vi "Teleop.vi"(10 "Match Info":T1={"Autonomous Elapsed Seconds"=0.0, "TeleOp Elapsed Seconds"=0.0, "Disabled Elapsed Seconds"=0.0, "Visited Autonomous"=FALSE, "Visited TeleOp"=FALSE, "Visited Disabled"=FALSE, "Autonomous Settings"={"Autonomous Style"=enum."Independent", "VI Refnum"=refnum}}, 11 "Call Context":T2) -> ()   [LabVIEW 2015]
doc: "This VI is called for each TeleOp packet received from the DS where the robot is not disabled. It is often used to read from the joysticks and update I/O or to update setpoints for timed control loops. It should complete and return within 20 milliseconds or it may miss DS packets."
uses:
  <vilib>/Rock Robotics/WPI/DriverStation/WPI_DriverStationDerivedRobotMode.ctl
  <vilib>/Rock Robotics/WPI/DriverStation/WPI_DriverStationMatch Info.ctl
  <vilib>/Rock Robotics/WPI/Utilities/WPI_GetSetVariantRefNum.vi
  Robot Global Data.vi
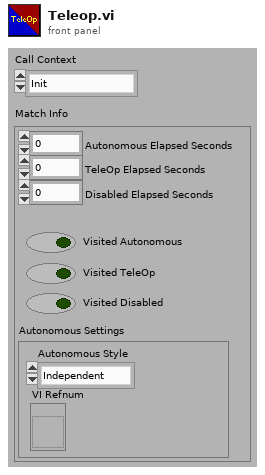
[diagram p1: front panel]
types:
  T1 = typedef "WPI_DriverStationMatch Info.ctl" = cluster{"Autonomous Elapsed Seconds":dbl, "TeleOp Elapsed Seconds":dbl, "Disabled Elapsed Seconds":dbl, "Visited Autonomous":bool, "Visited TeleOp":bool, "Visited Disabled":bool, "Autonomous Settings":cluster{"Autonomous Style":enum16{"Iterative", "Independent"}, "VI Refnum":refnum<vi>}}
  T2 = typedef "WPI_DriverStationDerivedRobotMode.ctl" = enum16{"Init", "Execute", "Stop"}
  T3 = typedef "WPI_JoystickDevRef.ctl" = cluster{"Device":T4}
  T4 = typedef "WPI_JoystickDeviceEnum.ctl" = enum16{"USB 0", "USB 1", "USB 2", "USB 3", "USB 4", "USB 5"}
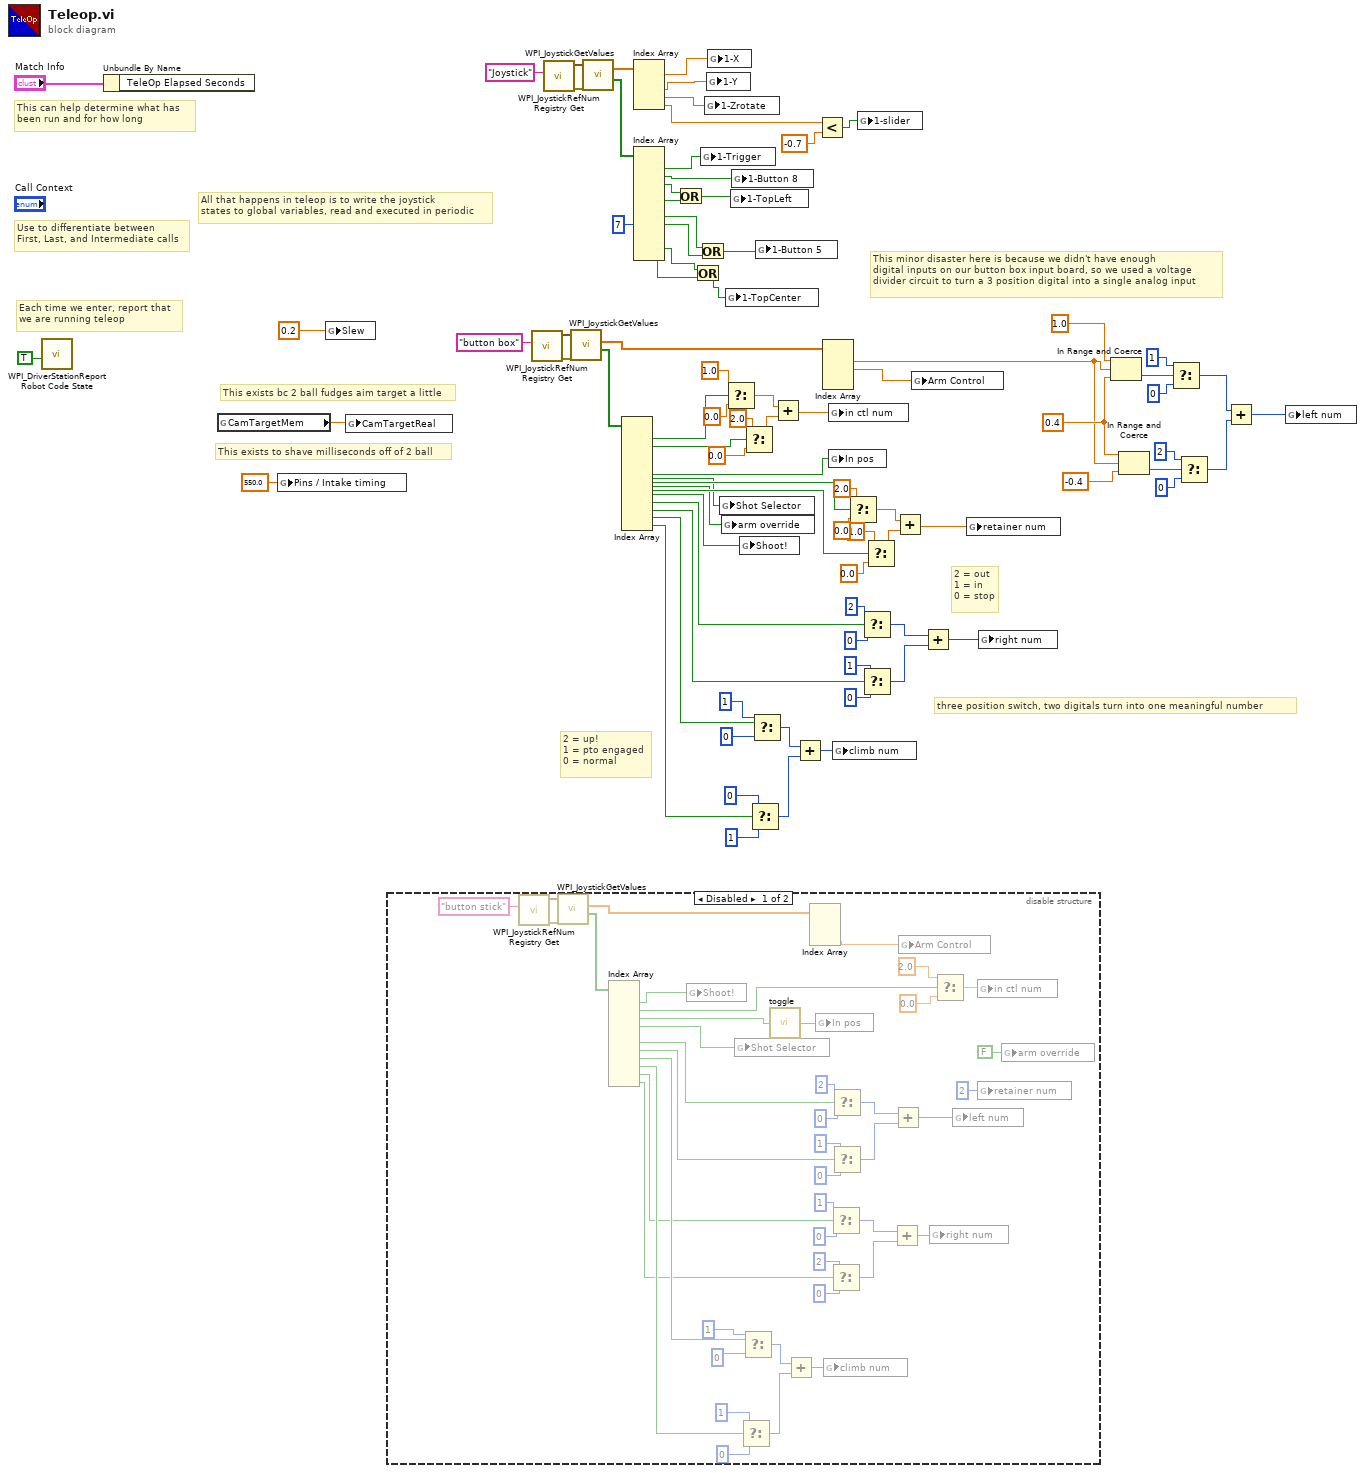
[diagram p0: block diagram]
diagram:
  w31 = 0.4 ("upper limit")
  # "three position switch, two digitals turn into one meaningful number"
  # "This minor disaster here is because we didn't have enough\ndigital inputs on our button box input board, so we used a voltage\ndivider circuit to turn a 3 position digital into a single analog input"
  # "This exists to shave milliseconds off of 2 ball"
  # "This exists bc 2 ball fudges aim target a little"
  # "All that happens in teleop is to write the joystick\nstates to global variables, read and executed in periodic"
  # "2 = up!\n1 = pto engaged\n0 = normal"
  # "2 = out\n1 = in\n0 = stop"
  # "Each time we enter, report that\nwe are running teleop"
  # "Use to differentiate between\nFirst, Last, and Intermediate calls"
  # "This can help determine what has\nbeen run and for how long"
  n1 = call <vilib>:"WPI_DriverStationReport Robot Code State.vi"("TeleOp"=TRUE ("Autonomous")) -> ()  [unwired: 10 in, 1 out]
  n2 = Unbundle By Name("Match Info") -> ()  [unwired: 1 out]
  n3 = global read "Robot Global Data.vi" "CamTargetMem"() -> (w1:dbl)
  n4 = global write "Robot Global Data.vi" "Pins / Intake timing"(550.0 ("Pins / Intake timing")) -> ()
  n5 = global write "Robot Global Data.vi" "Slew"(0.2 ("PTO speed")) -> ()
  n6 = global write "Robot Global Data.vi" "CamTargetReal"(w1) -> ()
  n7 = disable-structure shown="Disabled" {
    frame Disabled {
      n8 = call <vilib>:"WPI_JoystickRefNum Registry Get.vi"("refnum name"="button stick") -> ("error out"=w129:errorcluster, "JoystickDevRef"=w128:T3)  [unwired: 9 in]
      n9 = call <vilib>:"WPI_JoystickGetValues.vi"("error in (no error)"=w129, "JoystickDevRef"=w128) -> ("Buttons"=w127:bool[], "Axes"=w121:dbl[])  [unwired: 5 in, 3 out]
      n10 = Index Array(array=w127) -> (element #1=w110:bool, element #2=w106:bool, element #3=w104:bool, element #4=w101:bool, element #6=w93:bool, element #7=w92:bool, element #8=w91:bool, element #9=w90:bool, element #10=w89:bool, element #11=w88:bool)  [unwired: 11 in, 1 out]
      n11 = global write "Robot Global Data.vi" "Shoot!"(w110) -> ()
      n12 = global write "Robot Global Data.vi" "Shot Selector"(w101) -> ()
      n13 = Select(t=1, s=w90, f=0) -> (s? t:f=w118:i32)
      n14 = Select(t=1, s=w91, f=0) -> (s? t:f=w117:i32)
      n15 = call "toggle.vi"("Input"=w104) -> ("Output"=w105:bool)
      n16 = Add(x=w117, y=w118) -> (x+y=w116:i32)
      n17 = Index Array(array=w121) -> (element #3=w111:dbl)  [unwired: 3 in, 2 out]
      n18 = global write "Robot Global Data.vi" "In pos"(w105) -> ()
      n19 = global write "Robot Global Data.vi" "climb num"(w116) -> ()
      n20 = Select(t=i8 1, s=w89, f=i8 0) -> (s? t:f=w97:i8)
      n21 = Select(t=i8 2, s=w88, f=i8 0) -> (s? t:f=w98:i8)
      n22 = Select(t=i8 2, s=w93, f=i8 0) -> (s? t:f=w123:i8)
      n23 = Select(t=i8 1, s=w92, f=i8 0) -> (s? t:f=w124:i8)
      n24 = Add(x=w97, y=w98) -> (x+y=w94:i8)
      n25 = Add(x=w123, y=w124) -> (x+y=w122:i8)
      n26 = global write "Robot Global Data.vi" "Arm Control"(w111) -> ()
      n27 = global write "Robot Global Data.vi" "right num"(w94) -> ()
      n28 = Select(t=2.0, s=w106, f=0.0) -> (s? t:f=w107:dbl)
      n29 = global write "Robot Global Data.vi" "left num"(w122) -> ()
      n30 = global write "Robot Global Data.vi" "in ctl num"(w107) -> ()
      n31 = global write "Robot Global Data.vi" "retainer num"(i16 2 ("retainer num")) -> ()
      n32 = global write "Robot Global Data.vi" "arm override"(FALSE ("arm override")) -> ()
    }
    frame Enabled {
    }
  }
  n33 = call <vilib>:"WPI_JoystickRefNum Registry Get.vi"("refnum name"="button box") -> ("error out"=w74:errorcluster, "JoystickDevRef"=w73:T3)  [unwired: 9 in]
  n34 = call <vilib>:"WPI_JoystickRefNum Registry Get.vi"("refnum name"="Joystick") -> ("error out"=w84:errorcluster, "JoystickDevRef"=w83:T3)  [unwired: 9 in]
  n35 = call <vilib>:"WPI_JoystickGetValues.vi"("error in (no error)"=w74, "JoystickDevRef"=w73) -> ("Buttons"=w72:bool[], "Axes"=w46:dbl[])  [unwired: 5 in, 3 out]
  n36 = call <vilib>:"WPI_JoystickGetValues.vi"("error in (no error)"=w84, "JoystickDevRef"=w83) -> ("Buttons"=w80:bool[], "Axes"=w82:dbl[])  [unwired: 5 in, 3 out]
  n37 = Index Array(array=w72) -> (element #1=w65:bool, element #2=w64:bool, element #3=w63:bool, element #4=w58:bool, element #5=w57:bool, element #6=w56:bool, element #7=w55:bool, element #8=w54:bool, element #9=w48:bool, element #10=w47:bool, element #11=w40:bool, element #12=w39:bool)  [unwired: 12 in]
  n38 = Index Array(array=w82) -> (element #1=w77:dbl, element #2=w78:dbl, element #3=w81:dbl, element #4=w4:dbl)  [unwired: 4 in]
  n39 = Index Array(array=w80, index #8=7 ("index")) -> (element #1=w79:bool, element #2=w16:bool, element #3=w14:bool, element #5=w13:bool, element #7=w12:bool, element #8=w11:bool, element #11=w9:bool, element #12=w8:bool)  [unwired: 11 in, 4 out]
  n40 = Or(x=w14, y=w13) -> (x .or. y?=w15:bool)
  n41 = Or(x=w9, y=w8) -> (x .or. y?=w7:bool)
  n42 = Or(x=w12, y=w11) -> (x .or. y?=w10:bool)
  n43 = global write "Robot Global Data.vi" "1-Trigger"(w79) -> ()
  n44 = global write "Robot Global Data.vi" "1-Zrotate"(w81) -> ()
  n45 = global write "Robot Global Data.vi" "1-Y"(w78) -> ()
  n46 = global write "Robot Global Data.vi" "1-X"(w77) -> ()
  n47 = global write "Robot Global Data.vi" "Shot Selector"(w56) -> ()
  n48 = global write "Robot Global Data.vi" "arm override"(w55) -> ()
  n49 = global write "Robot Global Data.vi" "1-TopCenter"(w7) -> ()
  n50 = Select(t=1.0, s=w65, f=0.0) -> (s? t:f=w67:dbl)
  n51 = global write "Robot Global Data.vi" "1-TopLeft"(w15) -> ()
  n52 = global write "Robot Global Data.vi" "1-Button 8"(w16) -> ()
  n53 = global write "Robot Global Data.vi" "Shoot!"(w54) -> ()
  n54 = Select(t=2.0, s=w64, f=0.0) -> (s? t:f=w68:dbl)
  n55 = Select(t=0, s=w39, f=1) -> (s? t:f=w43:i32)
  n56 = Select(t=1, s=w40, f=0) -> (s? t:f=w42:i32)
  n57 = global write "Robot Global Data.vi" "1-Button 5"(w10) -> ()
  n58 = Add(x=w67, y=w68) -> (x+y=w66:dbl)
  n59 = Add(x=w42, y=w43) -> (x+y=w41:i32)
  n60 = Less?(x=w4, y=-0.7) -> (x < y?=w6:bool)
  n61 = Index Array(array=w46) -> (element #1=w28:dbl, element #2=w38:dbl)  [unwired: 4 in, 2 out]
  n62 = global write "Robot Global Data.vi" "in ctl num"(w66) -> ()
  n63 = global write "Robot Global Data.vi" "In pos"(w63) -> ()
  n64 = global write "Robot Global Data.vi" "climb num"(w41) -> ()
  n65 = Select(t=2.0, s=w58, f=0.0) -> (s? t:f=w60:dbl)
  n66 = global write "Robot Global Data.vi" "1-slider"(w6) -> ()
  n67 = Select(t=i8 2, s=w48, f=i8 0) -> (s? t:f=w50:i8)
  n68 = Select(t=i8 1, s=w47, f=i8 0) -> (s? t:f=w51:i8)
  n69 = Select(t=1.0, s=w57, f=0.0) -> (s? t:f=w61:dbl)
  n70 = Add(x=w60, y=w61) -> (x+y=w59:dbl)
  n71 = global write "Robot Global Data.vi" "Arm Control"(w38) -> ()
  n72 = Add(x=w50, y=w51) -> (x+y=w49:i8)
  n73 = global write "Robot Global Data.vi" "retainer num"(w59) -> ()
  n74 = global write "Robot Global Data.vi" "right num"(w49) -> ()
  n75 = In Range and Coerce(upper limit=1.0, x=w28, lower limit=w31) -> (In Range?=w34:bool)  [unwired: 1 out]
  n76 = In Range and Coerce(upper limit=w31, x=w28, lower limit=-0.4) -> (In Range?=w37:bool)  [unwired: 1 out]
  n77 = Select(t=i8 1, s=w34, f=i8 0) -> (s? t:f=w27:i8)
  n78 = Select(t=i8 2, s=w37, f=i8 0) -> (s? t:f=w26:i8)
  n79 = Add(x=w27, y=w26) -> (x+y=w17:i8)
  n80 = global write "Robot Global Data.vi" "left num"(w17) -> ()
